vi "Write PS Channel.vi"(8 "error in (no error)":errorcluster, 10 "PS Channel":T1, 11 "PS Channel configuration":refnum<class "Power Supply Channel configuration.lvclass">) -> (0 "error out":errorcluster, 3 "PS Channel configuration out":refnum<class "Power Supply Channel configuration.lvclass">)   [LabVIEW 2025, in "Power Supply.lvlib" / "Power Supply Channel configuration.lvclass"]
uses:
  Power Supply Channel configuration.lvclass
  PS Channel Setting.ctl
  Power Supply Channel configuration.lvclass/Power Supply Channel configuration.ctl
panel:
  # "Output Control"
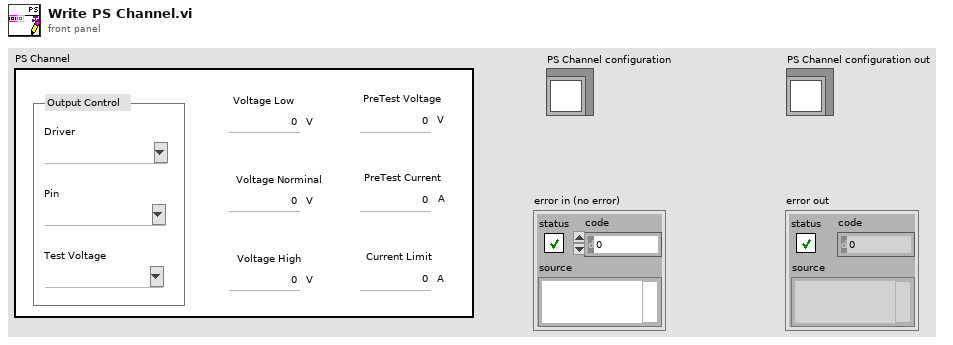
[diagram p1: front panel]
types:
  T1 = typedef "Power Supply.lvlib/Power Supply Channel configuration.lvclass/PS Channel Setting.ctl" = cluster{"Driver":string, "Pin":string, "Test Voltage":string, "Voltage Low":dbl, "Voltage Norminal":dbl, "Voltage High":dbl, "PreTest Voltage":dbl, "PreTest Current":dbl, "Current Limit":dbl}
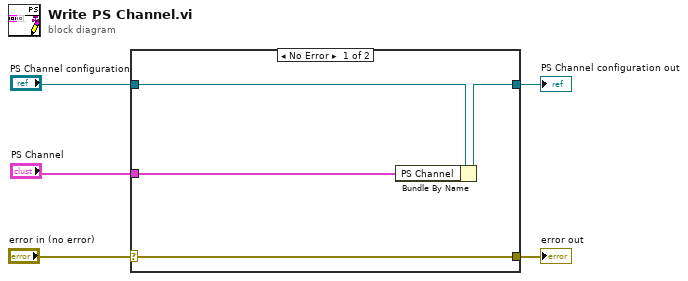
[diagram p0: block diagram]
diagram:
  n1 = case shown="No Error" "error in (no error)" {
    selector: "error in (no error)" -> [w9 w10]
    tunnel: [w9 w10] -> w4
    tunnel: [w7 w11] -> w2
    tunnel: "PS Channel configuration" -> [w8 w11]
    tunnel: "PS Channel" -> [w6 _]
    frame No Error {
      n2 = Bundle By Name(cluster=w8, "PS Channel"=w6) -> (w7:refnum<class "Power Supply Channel configuration.lvclass">)
    }
    frame Error {
    }
  }
  "error out" <- w4
  "PS Channel configuration out" <- w2
